vi "wait_for_stim.vi"(4 "vars in":T1={"wait count t"=0, "wait min"=0, "wait max"=0, "stim count t"=0, "stim count n"=0, "d stim"=0, "d timeout"=0, "timeout win"=0, "base temp"=0.0, "stim amps"=[], "n hit"=0, "n catch"=0, "active"=TRUE, "catch"=TRUE, "stimulus"=TRUE, "reward given"=TRUE, "pairing"=TRUE, "lick"=FALSE, "next reward"=FALSE, "clean tubes"=FALSE, "next temp"=0.0}) -> (1 "vars out":T1={"wait count t"=0, "wait min"=0, "wait max"=0, "stim count t"=0, "stim count n"=0, "d stim"=0, "d timeout"=0, "timeout win"=0, "base temp"=0.0, "stim amps"=[], "n hit"=0, "n catch"=0, "active"=TRUE, "catch"=TRUE, "stimulus"=TRUE, "reward given"=TRUE, "pairing"=TRUE, "lick"=FALSE, "next reward"=FALSE, "clean tubes"=FALSE, "next temp"=0.0})   [LabVIEW 2015]
uses:
  Type Definitions/vars.ctl
panel:
  # "(see Block Diagram)"
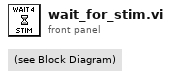
[diagram p1: front panel]
types:
  T1 = typedef "vars.ctl" = cluster{"wait count t":u16, "wait min":u16, "wait max":u16, "stim count t":u16, "stim count n":u16, "d stim":u16, "d timeout":u16, "timeout win":u16, "base temp":sgl, "stim amps":i32[], "n hit":u16, "n catch":u16, "active":bool, "catch":bool, "stimulus":bool, "reward given":bool, "pairing":bool, "lick":bool, "next reward":bool, "clean tubes":bool, "next temp":sgl}
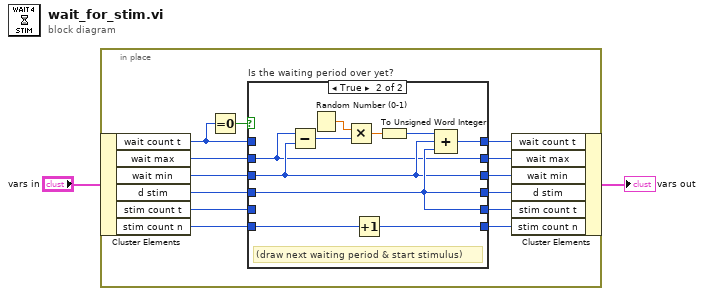
[diagram p0: block diagram]
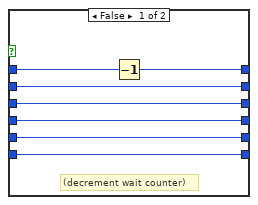
[diagram p2: hidden frame]
diagram:
  n1 = in-place {
    n2 = in-place-cluster #1("vars in") -> ("wait count t"=w12:u16, "wait max"=w11:u16, "wait min"=w10:u16, "d stim"=w9:u16, "stim count t"=w8:u16, "stim count n"=w14:u16)
    n3 = Equal To 0?(x=w12) -> (x = 0?=w15:bool)
    n4 = case "Is the waiting period over yet?" shown="True" w15 {
      tunnel: w12 -> [w22 _]
      tunnel: [w21 w23] -> w7
      tunnel: w11 -> [w18 w26]
      tunnel: w10 -> [w19 w27]
      tunnel: w9 -> [w20 w28]
      tunnel: w8 -> [w17 _]
      tunnel: w14 -> [w16 w32]
      tunnel: [w16 w31] -> w13
      tunnel: [w17 w28] -> w6
      tunnel: [w20 w28] -> w5
      tunnel: [w19 w27] -> w4
      tunnel: [w18 w26] -> w3
      frame False {
        # "(decrement wait counter)"
        n5 = Decrement(x=w22) -> (x-1=w21:u16)
      }
      frame True {
        # "(draw next waiting period & start stimulus)"
        n6 = Subtract(x=w26, y=w27) -> (x-y=w30:u16)
        n7 = Random Number (0-1)() -> (number: 0 to 1=w29:dbl)
        n8 = Multiply(x=w29, y=w30) -> (x*y=w25:dbl)
        n9 = Increment(x=w32) -> (x+1=w31:u16)
        n10 = To Unsigned Word Integer(number=w25) -> (unsigned 16bit integer=w24:u16)
        n11 = Compound Arithmetic op=ADD(w24, w27, w28) -> (w23:u16)
      }
    }
    n12 = in-place-cluster #1("wait count t"=w7, "wait max"=w3, "wait min"=w4, "d stim"=w5, "stim count t"=w6, "stim count n"=w13) -> (→"vars out":T1)
  }
